vi "Comparison.vi"(8 "error in (no error)":errorcluster, 10 "Level":dbl, 11 "Aim Middle Threshold in":refnum<class "Aim Middle Threshold.lvclass">) -> (0 "error out":errorcluster, 2 "Color":u32(colorbox))   [LabVIEW 2021, in "Aim Middle Threshold.lvclass"]
uses:
  Aim Middle Threshold.lvclass
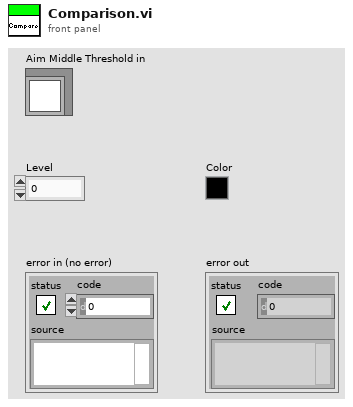
[diagram p1: front panel]
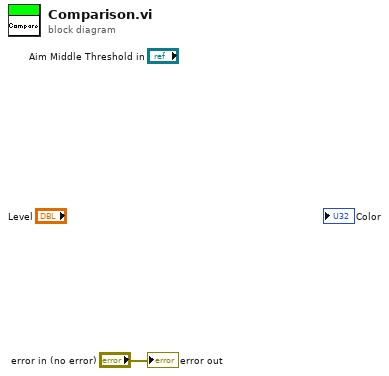
[diagram p0: block diagram]
diagram:
  "error out" <- "error in (no error)"
